vi "Write UI Manipulation CMD.vi"(8 "error in (no error)":errorcluster, 10 "UI Manipulation CMD":i64, 11 "UI Console MSG in":refnum<class "UI Console MSG.lvclass">) -> (0 "error out":errorcluster, 3 "UI Console MSG out":refnum<class "UI Console MSG.lvclass">)   [LabVIEW 2024, in "UI Console MSG.lvclass"]
uses:
  UI Console MSG.lvclass
  UI Console MSG.lvclass/UI Console MSG.ctl
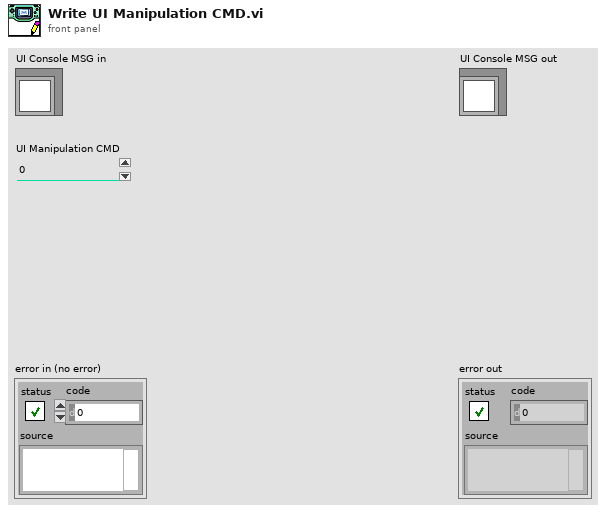
[diagram p1: front panel]
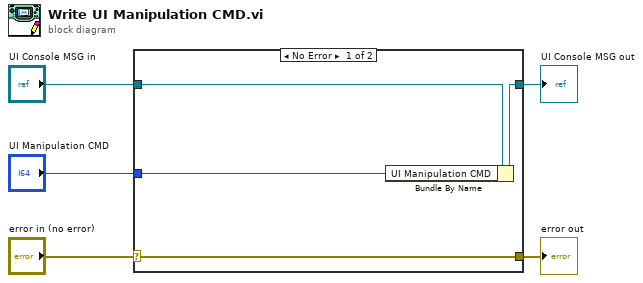
[diagram p0: block diagram]
diagram:
  n1 = case shown="No Error" "error in (no error)" {
    selector: "error in (no error)" -> [w9 w10]
    tunnel: [w9 w10] -> w4
    tunnel: [w7 w11] -> w2
    tunnel: "UI Console MSG in" -> [w8 w11]
    tunnel: "UI Manipulation CMD" -> [w6 _]
    frame No Error {
      n2 = Bundle By Name(cluster=w8, "UI Manipulation CMD"=w6) -> (w7:refnum<class "UI Console MSG.lvclass">)
    }
    frame Error {
    }
  }
  "error out" <- w4
  "UI Console MSG out" <- w2
